vi "Create Temp File.vi"(8 "Error In":errorcluster, 11 "Settings Filepath":path) -> (0 "Error Out":errorcluster, 3 "Temp Settings Filepath":path)   [LabVIEW 2023, in "Error Manager.lvlib" / "Settings.lvclass"]
doc: "This VI creates a temporary copy of the Error Manager settings file. Operations such as removing comments will be performed on the temp file. This ensures that the original settings file is left unchanged. The temp file will be deleted shortly after."
uses:
  Settings.lvclass
  Settings.lvclass/Settings.ctl
panel:
  # "Development\nControls or indicators that are useful for development or testing, but which are not outputs of the VI."
  # "Input\nInputs to the VI"
  # "Output\nOutputs of the VI"
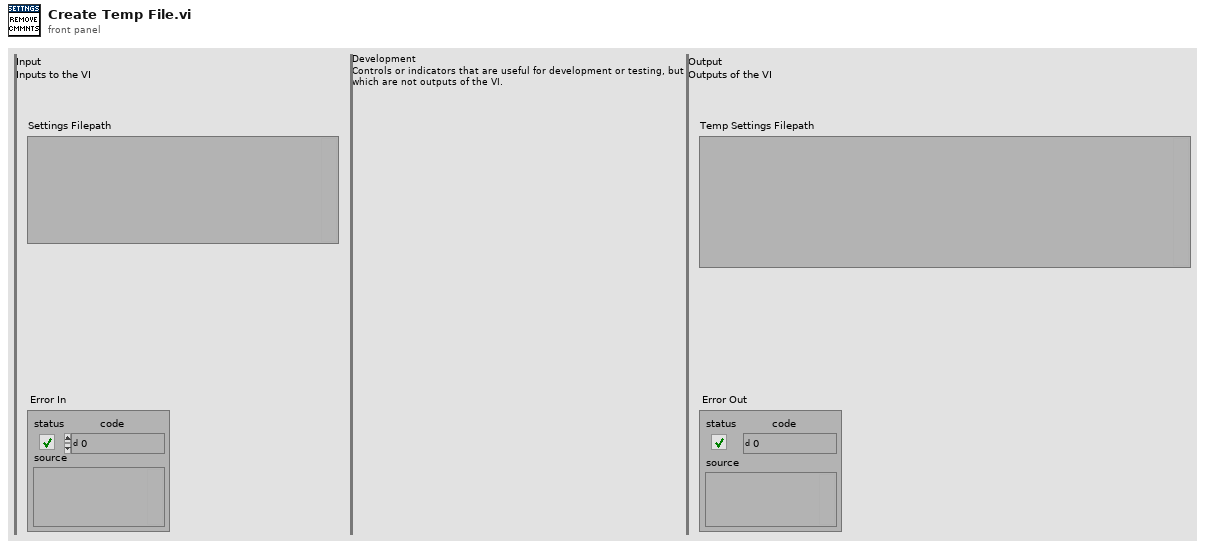
[diagram p1: front panel]
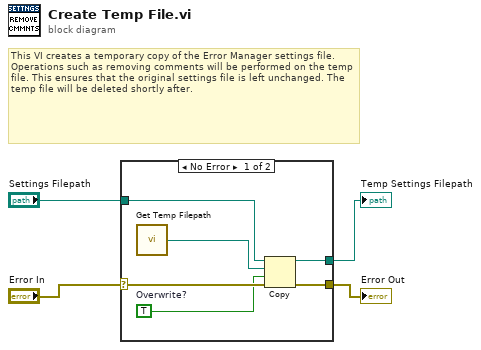
[diagram p0: block diagram]
diagram:
  # "This VI creates a temporary copy of the Error Manager settings file. Operations such as removing comments will be performed on the temp file. This ensures that the original settings file is left unchanged. The temp file will be deleted shortly after."
  n1 = case shown="No Error" "Error In" {
    selector: "Error In" -> [w10 w11]
    tunnel: [w9 w11] -> w3
    tunnel: "Settings Filepath" -> [w8 _]
    tunnel: [w5 _] -> w1
    frame No Error {
      w7 = TRUE  # Overwrite?
      n2 = call "Get Temp Filepath.vi"() -> ("Temp Settings Filepath"=w6:path)
      n3 = Copy(8:w10, 9:w7, 10:w6, 11:w8) -> (0:w9:errorcluster, 3:w5:path)  [unwired: 1 in, 1 out]
    }
    frame Error {
    }
  }
  "Error Out" <- w3
  "Temp Settings Filepath" <- w1
